vi "cmdmain.vi"(11 "command line arguments":T1) -> (0 "error out":errorcluster)   [LabVIEW 2013]
uses:
  arguments.ctl
  <vilib>/Utility/sysdir.llb/Get System Directory.vi
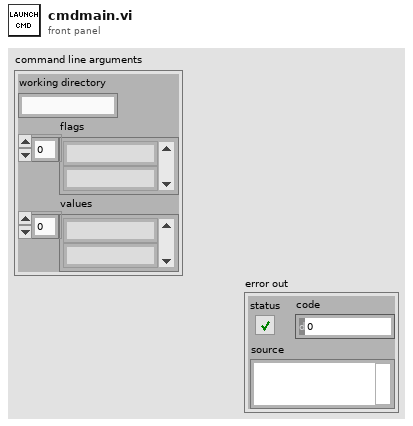
[diagram p1: front panel]
types:
  T1 = typedef "arguments.ctl" = cluster{"working directory":string, "flags":string[], "values":string[]}
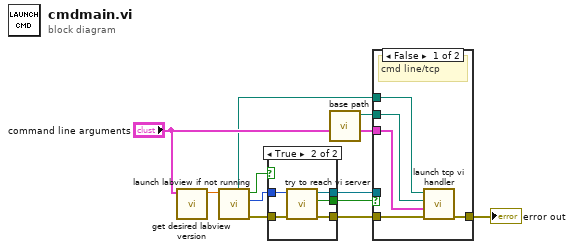
[diagram p0: block diagram]
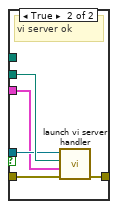
[diagram p2: hidden frame]
diagram:
  n1 = call "get desired labview version.vi"("command line arguments"="command line arguments") -> ("lv version"=w2:dbl)  [unwired: 10 in]
  n2 = call "launch labview if not running.vi"("desired lv version"=w2) -> ("error out"=w10:errorcluster, "port"=w9:u32, "vi server available"=w11:bool, "labview directory"=w1:path)  [unwired: 6 in, 1 out]
  n3 = case shown="True" w11 {
    selector: w11 -> [w12 _]
    tunnel: w10 -> [w13 w17]
    tunnel: w9 -> [_ w18]
    tunnel: [w13 w14] -> w6
    tunnel: [w12 w15] -> w8
    tunnel: [_ w16] -> w7
    frame False {
    }
    frame True {
      n4 = call "try to reach vi server.vi"("error in"=w17, "port"=w18) -> ("error out"=w14:errorcluster, "connected"=w15:bool, "Application out"=w16:refnum<vi>)  [unwired: 7 in]
    }
  }
  n5 = call "base path.vi"() -> ("base path"=w4:path)  [unwired: 11 in]
  n6 = case shown="False" w8 {
    tunnel: w7 -> [_ w26]
    tunnel: w4 -> [w23 w28]
    tunnel: w6 -> [w19 w27]
    tunnel: "command line arguments" -> [w22 w25]
    tunnel: [w21 w24] -> w5
    tunnel: w1 -> [w20 _]
    frame False {
      # "cmd line/tcp"
      n7 = call "launch tcp vi handler.vi"("error in"=w19, "command line arguments"=w22, "base path"=w23, "labview directory"=w20) -> ("error out"=w21:errorcluster)  [unwired: 7 in]
    }
    frame True {
      # "vi server ok"
      n8 = call "launch vi server handler.vi"("error in"=w27, "command line arguments"=w25, "base path"=w28, "Application in"=w26) -> ("error out"=w24:errorcluster)  [unwired: 7 in]
    }
  }
  "error out" <- w5
